vi "Turning with time.vi"(8 "error in (no error)":errorcluster, 11 "Turn? Right Positive.":dbl) -> (0 "error out":errorcluster)   [LabVIEW 2017]
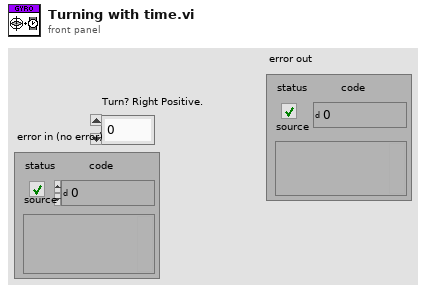
[diagram p1: front panel]
types:
  T1 = typedef "DriveMotors.ctl" = cluster{"MotorControlDevRef":T2, "MotorControlDevRef":T2, "MotorControlDevRef":T2, "MotorControlDevRef":T2, "MotorControlDevRef":T2, "MotorControlDevRef":T2}
  T2 = typedef "WPI_MotorControlDeviceRef.ctl" = cluster{"DeviceStatus":errorcluster, "Type":T3, "PWM":cluster{"PWM Channel":T4, "DeadBand":T5}, "CAN":cluster{"Device Number":u8, "SetOutput VI Ref":variant, "GetOutput VI Ref":variant, "Enable VI Ref":variant, "Disable VI Ref":variant, "Data":variant}, "Invert":bool, "DIO PWM":cluster{"PWM \"Enable\" Channel":T4, "DIOChannel":T6, "PWM Rate":dbl}}
  T3 = typedef "WPI_MotorControlType.ctl" = enum16{"PWM", "CAN", "DIO PWM"}
  T4 = typedef "FPGA_DIOPWMChannel.ctl" = enum8{"PWM 0", "PWM 1", "PWM 2", "PWM 3", "PWM 4", "PWM 5", "PWM 6", "PWM 7", "PWM 8", "PWM 9", "PWM MXP 0", "PWM MXP 1", "PWM MXP 2", "PWM MXP 3", "PWM MXP 4", "PWM MXP 5", "PWM MXP 6", "PWM MXP 7", "PWM MXP 8", "PWM MXP 9", "Invalid"}
  T5 = typedef "WPI_PWMDeadband.ctl" = cluster{"Name":string, "maxPositivePwm":i32, "minPositivePwm":i32, "centerPwm":i32, "maxNegativePwm":i32, "minNegativePwm":i32, "angularRange":u16}
  T6 = typedef "FPGA_DIOChannel.ctl" = enum8{"DIO 0", "DIO 1", "DIO 2", "DIO 3", "DIO 4", "DIO 5", "DIO 6", "DIO 7", "DIO 8", "DIO 9", "DIO MXP 0", "DIO MXP 1", "DIO MXP 2", "DIO MXP 3", "DIO MXP 4", "DIO MXP 5", "DIO MXP 6", "DIO MXP 7", "DIO MXP 8", "DIO MXP 9", "DIO MXP 10", "DIO MXP 11", "DIO MXP 12", "DIO MXP 13", "DIO MXP 14", "DIO MXP 15", "SPI Port CS1", "SPI Port CS2", "SPI Port CS3", "SPI Port MISO", "SPI Port MOSI", "Invalid"}
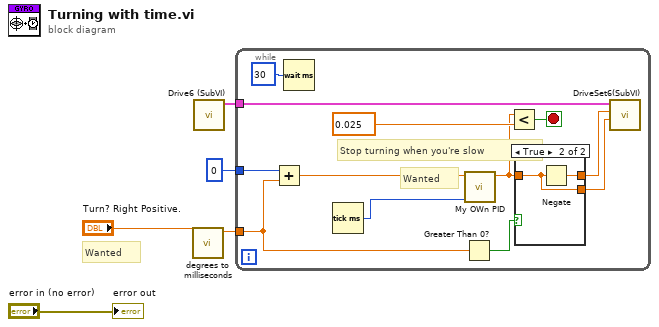
[diagram p0: block diagram]
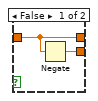
[diagram p2: hidden frame]
diagram:
  # "Wanted"
  n1 = call "degrees to milliseconds.vi"("Distance in feet wanted"="Turn? Right Positive.") -> ("milliseconds"=w2:dbl)  [unwired: 10 in]
  n2 = call "Drive6 (SubVI).vi"() -> ("DriveControlDevRef"=w5:T1)  [unwired: 11 in]
  n3 = while {
    tunnel: w2 -> [w8]
    tunnel: w5 -> [w10]
    tunnel: 0 -> [w7]
    stop <- w15 stop-if-true
    # "Wanted"
    # "Stop turning when you're slow"
    n4 = Add(x=w7, y=w8) -> (x+y=w9:dbl)
    n5 = Wait (ms)(milliseconds to wait=u32 30) -> ()  [unwired: 1 out]
    n6 = Tick Count (ms)() -> (millisecond timer value=w6:u32)
    n7 = Greater Than 0?(x=w8) -> (x > 0?=w14:bool)
    n8 = call "My OWn PID.vi"("Current Input"=w6, "Wanted End"=w9) -> ("Output"=w13:dbl)  [unwired: 9 in]
    n9 = Less?(x=w13, y=0.025) -> (x < y?=w15:bool)
    n10 = case shown="True" w14 {
      tunnel: w13 -> [w18 w20]
      tunnel: [w18 w21] -> w12
      tunnel: [w19 w20] -> w11
      frame False {
        n11 = Negate(x=w18) -> (-x=w19:dbl)
      }
      frame True {
        n12 = Negate(x=w20) -> (-x=w21:dbl)
      }
    }
    n13 = call "DriveSet6(SubVI).vi"("Left"=w11, "Right"=w12, "output cluster"=w10) -> ()  [unwired: 8 in, 1 out]
  }
  "error out" <- "error in (no error)"
